vi "RP_Version.vi"(8 "error in (no error)":errorcluster) -> (0 "error out":errorcluster, 3 "REFPROP Version Number":string)   [LabVIEW 2015]
doc: "Returns the REFPROP dll version number."
uses:
  REFPROP.dll
panel:
  # "REFPROP-RP_VERSION.vi"
  # "void  RPVersion(CStr Version, int32_t length);"
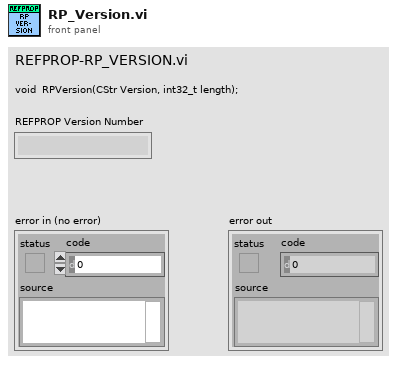
[diagram p1: front panel]
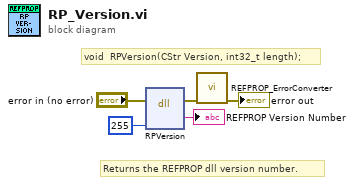
[diagram p0: block diagram]
diagram:
  # "void  RPVersion(CStr Version, int32_t length);"
  # "Returns the REFPROP dll version number."
  n1 = dll-call lib="C:/Users/lauria/Desktop/REFPROP 10 LabVIEW Wrapper BETA/REFPROP/REFPROP.*" fn="RPVersion"(error in="error in (no error)", "length"=255 ("ln")) -> (error out=w3:errorcluster, "Version"=→"REFPROP Version Number":string)  [unwired: 5 in, 1 out]
  n2 = call "REFPROP_ErrorConverter.vi"("error in (no error)"=w3) -> ("error out"=→"error out":errorcluster)  [unwired: 10 in]
